vi "SolenoidA.vi"() -> (3 "Thermometer":dbl(slide) scale=140.0..170.0)   [LabVIEW 2018, in "com.Instrument.lvlib"]
uses:
  com.Instrument.lvlib
  global/Solenoid Temp.vi
panel:
  out "error out":errorcluster
  out "VISA resource name out":refnum<visa-resource-name>
  in  "error in (no error)":errorcluster
  in  "VISA resource name":refnum<visa-resource-name>
  in  "Serial Configuration":T1={"Baud Rate"=9600, "Parity"=0, "Data Bits"=8, "Flow Control"=4} {"Flow Control" items=["None", "XON/XOFF", "RTS/CTS", "XON/XOFF & RTS/CTS", "DTR/DSR", "XON/XOFF & DTR/DSR"]; "Data Bits" items=["7"=7, "8"=8]; "Parity" items=["None", "Odd", "Even", "Mark", "Space"]; "Baud Rate" items=["300"=300, "600"=600, "1200"=1200, "2400"=2400, "4800"=4800, "9600"=9600, "19200"=19200]}
  in  "Solenoid A Fake input":dbl(slide) scale=140.0..170.0
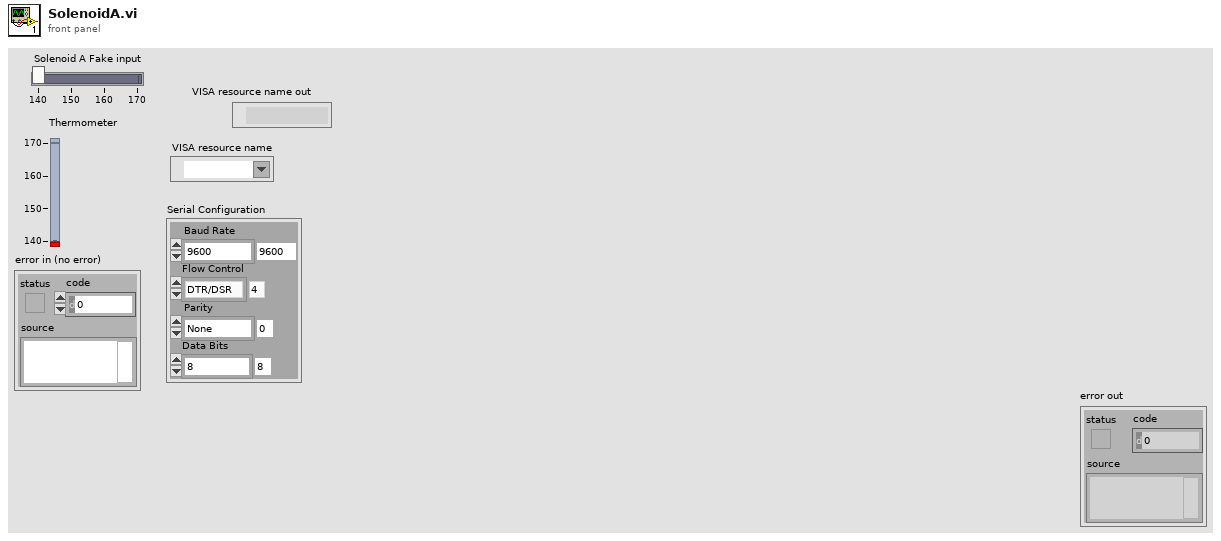
[diagram p1: front panel]
types:
  T1 = cluster{"Baud Rate":u32, "Parity":u16, "Data Bits":u16, "Flow Control":u16}
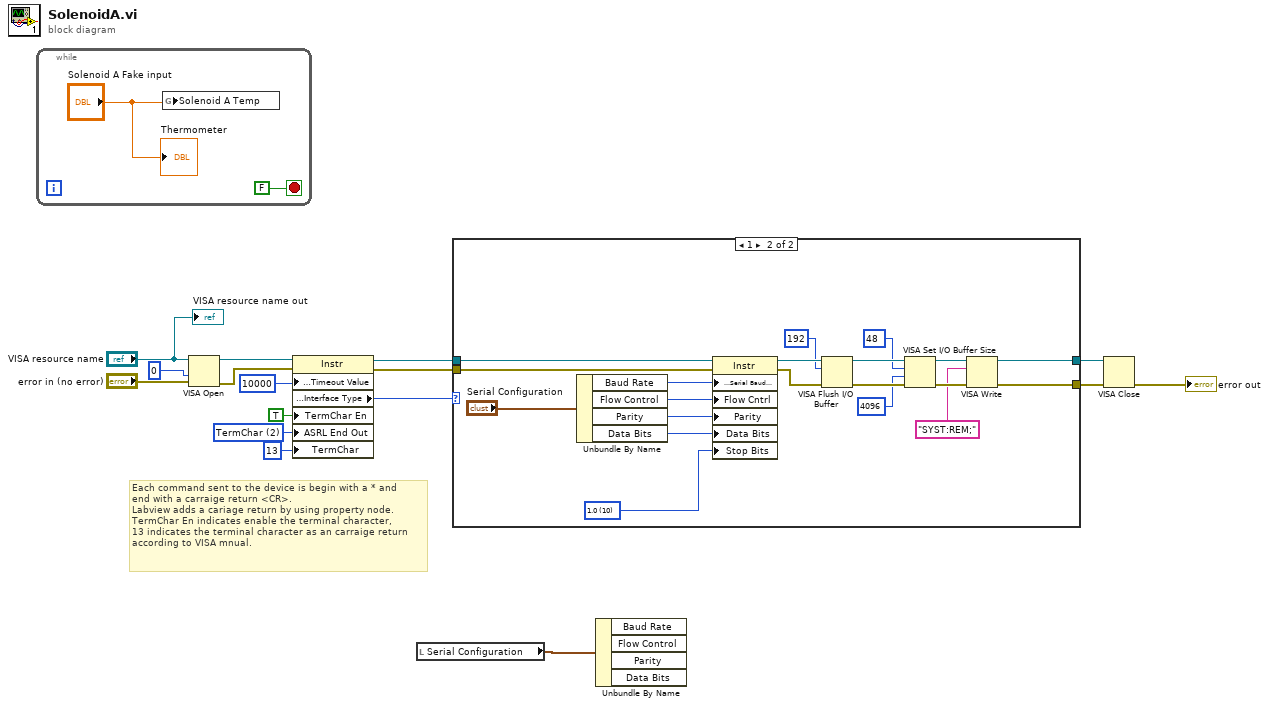
[diagram p0: block diagram]
diagram:
  w4 = u16 2 items=["None", "Last Bit", "TermChar", "Break"] ("Serial Settings:End Mode for Writes")
  # "Each command sent to the device is begin with a * and\nend with a carraige return <CR>.\nLabview adds a cariage return by using property node.\nTermChar En indicates enable the terminal character, \n13 indicates the terminal character as an carraige return \naccording to VISA mnual."
  n1 = while {
    stop <- FALSE stop-if-true
    n2 = global write "Solenoid Temp.vi" "Solenoid A Temp"("Solenoid A Fake input") -> ()
    "Thermometer" <- "Solenoid A Fake input"
  }
  n3 = VISA Open(access mode=u32 0, error in (no error)="error in (no error)", VISA resource name="VISA resource name") -> (VISA resource name=w15:refnum<visa-resource-name>, error out=w14:errorcluster)  [unwired: 2 in]
  n4 = property class="Instr"(reference=w15, error in=w14, "General Settings:Timeout Value"=u32 10000, "TermChar En"=TRUE ("Message Based Settings:Termination Character Enable"), "ASRL End Out"=w4, "TermChar"=u8 13 ("Message Based Settings:Termination Character")) -> (reference out=w8:refnum<visa-resource-name>, error out=w10:errorcluster, "Interface Information:Interface Type"=w11:u16)
  n5 = local read "Serial Configuration"() -> (w1:T1)
  n6 = case shown="1" w11 {
    tunnel: w8 -> [w20 w27]
    tunnel: w10 -> [w19 w26]
    tunnel: [w20 w22] -> w6
    tunnel: [w19 w21] -> w5
    frame 0, Default {
    }
    frame 1 {
      w28 = u16 10 items=["1.0"=10, "1.5"=15, "2.0"=20] ("Serial Settings:Stop Bits")
      n7 = Unbundle By Name("Serial Configuration") -> ("Baud Rate"=w32:u32, "Flow Control"=w31:u16, "Parity"=w30:u16, "Data Bits"=w29:u16)
      n8 = property class="Instr"(reference=w27, error in=w26, "Serial Settings:Serial Baud Rate"=w32, "Flow Cntrl"=w31, "Parity"=w30, "Data Bits"=w29, "Stop Bits"=w28) -> (reference out=w36:refnum<visa-resource-name>, error out=w37:errorcluster)
      n9 = VISA Flush I/O Buffer(VISA resource name=w36, mask (16)=u16 192, error in (no error)=w37) -> (VISA resource name out=w39:refnum<visa-resource-name>, error out=w38:errorcluster)
      n10 = VISA Set I/O Buffer Size(VISA resource name=w39, mask (16)=u16 48, size (4096)=u32 4096 ("size (0)"), error in (no error)=w38) -> (VISA resource name out=w25:refnum<visa-resource-name>, error out=w24:errorcluster)
      n11 = VISA Write(VISA resource name=w25, write buffer="SYST:REM;", error in (no error)=w24) -> (VISA resource name out=w22:refnum<visa-resource-name>, error out=w21:errorcluster)  [unwired: 1 out]
    }
  }
  n12 = Unbundle By Name(w1) -> ()  [unwired: 4 out]
  n13 = VISA Close(VISA resource name=w6, error in (no error)=w5) -> (error out=→"error out":errorcluster)
  "VISA resource name out" <- "VISA resource name"
